vi "MICSD Telem Driver.vi"(0 "VISA Resource Name":refnum<visa-resource-name>="COM3", 1 "Command":T1, 2 "Function":T2(ring)=enum."Transceive (DN -> UP)", 3 "Parameters":string, 5 "error in (no error)":errorcluster, 6 "Target MICS ID":u32=1048576 step=1 format="%.0x", 7 "Transceive Delay mS":dbl=200.0 min=0.0 max=10000.0 step=1.0, 8 "EXID":u32=16773121 step=1 format="%.0x", 9 "CP_DATA IN":u8[](array[numeric]), 10 "RF_Channel":u8=3) -> (13 "CP_DATA OUT":u8[](array[numeric]), 14 "Response Token":string, 15 "Response Code":string, 16 "bChecksum Valid":bool, 17 "tChecksum Valid":bool, 18 "Data":string, 19 "error out":errorcluster)   [LabVIEW 2010]
uses:
  Typedef Command List.ctl
  <vilib>/Utility/file.llb/Write To Spreadsheet File (string).vi
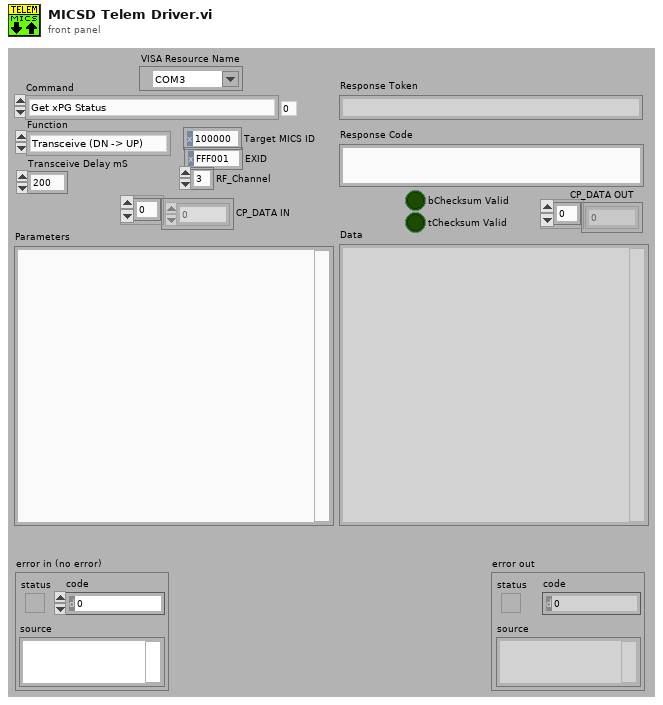
[diagram p1: front panel]
types:
  T1 = typedef "Typedef Command List.ctl" = enum16{"Get xPG Status", "xPG Stimulation", "Select Program", "Increment Program Amplitude", "Decrement Program Amplitude", "Get PoP Constants", "Get PPC Constants", "Get Program Names", "Set Pulse Amplitude", "Increment Pulse Amplitude", "Decrement Pulse Amplitude", "Get Pulse Widths", "Set Pulse Widths", "Increment Pulse Width", "Decrement Pulse Width", "Get Program Frequency", "Set Program Frequency", "Increment Program Frequency", "Decrement Program Frequency", "Inject Event", "Charging Control", "Get xPG Identity", "Set xPG Identity", "Restore Program Defaults", "Get Program Definition", "Set Program Definition", "Get Program Constants", "Set Program Constants", "Get Configurable Device Parameters", "Set Configurable Device Parameters", "Get Pulse Constants", "Set Pulse Constants", "Get Lead Limits", "Set Lead Limits", "Get Channel Calibrations", "Set Channel Calibrations", "<reserved 2>", "<reserved 3>", "<reserved 4>", "<reserved 5>", "<reserved 6>", "<reserved 7>", "Get Stim Asic HV Calibrations", "Set Stim Asic HV Calibrations", "<reserved 8>", "<reserved 9>", "Get CP Data", "Set CP Data", "Clear Log", "Read Log", "Append Log", "Get Patient Program Runtime", "Set Patient Program Runtime", "Impedance Measurement", "Enter Storage Mode", "Echo Short", "Echo Long", "Get General Calibration", "Set General Calibration", "Get Trim List", "Set Trim List", "Get Counter", "Set Counter", "Get Test Stimulation", "Set Test Stimulation", "Get Titration Stimulation", "Set Titration Stimulation", "Get Ramp Time", "Set Ramp Time", "Get VBAT", "Set Software Description Block", "Get Software Description Block", "Write Memory", "Read Memory", "Reset xPG", "Erase Flash Block", "Write Vectors", "Read Vectors", "Diagnostic Data", "Set Background Impedance", "Get Background Impedence ", "Set Test Waveform", "Calibrate Channel", "Get Log Range", "Reserved 0x55", "Reserved 0x56", "MICS Options", "Pair PPC", "Pair POP", "Stop Bootloader", "Tune MICS", "MICS Diagnostics", "Undefined"}
  T2 = enum16{"Open Session", "Close Session", "Downlink Only", "Uplink Only", "Transceive (DN -> UP)"}
  T3 = cluster{"ConfigFlags":u8, "ImplantID":u32, "CompanyID":u8, "Normal_Comm":cluster{"RF_Channel":u8, "UserData":u8, "TX_Mod":u8, "RX_Mod":u8, "RX_BlockSize":u8, "BlockPerPack":u8, "TX_BlockSize":u8}, "Emerg_Comm":cluster{"RF_Channel":u8, "UserData":u8, "TX_Mod":u8, "RX_Mod":u8, "TX_BlockSize":u8, "BlockPerPack":u8, "RX_BlockSize":u8}, "ImplantRev":u8, "245TX_PowerCal":i8, "245TX_Power":i8, "CCA_RSSI_Thresholds":cluster{"ch0":u16, "ch1":u16, "ch2":u16, "ch3":u16, "ch4":u16, "ch5":u16, "ch6":u16, "ch7":u16, "ch8":u16, "ch9":u16}}
  T4 = cluster{"ERROR_OCCURRED":bool, "LINK_STAT_CHANGED":bool, "LINK_QUAL_CHANGED":bool, "400MHZ_TX_ACTIVE":bool, "400MHZ_RX_ACTIVE":bool, "245GHZ_TX_ACTIVE":bool, "DATA_STAT_CHANGED":bool, "SLEEPING":bool, "IDLE":bool, "SEARCHING_FOR_IMPLANT":bool, "STARTING_SESSION":bool, "LISTENING_FOR_EMERG":bool, "IN_SESSION":bool}
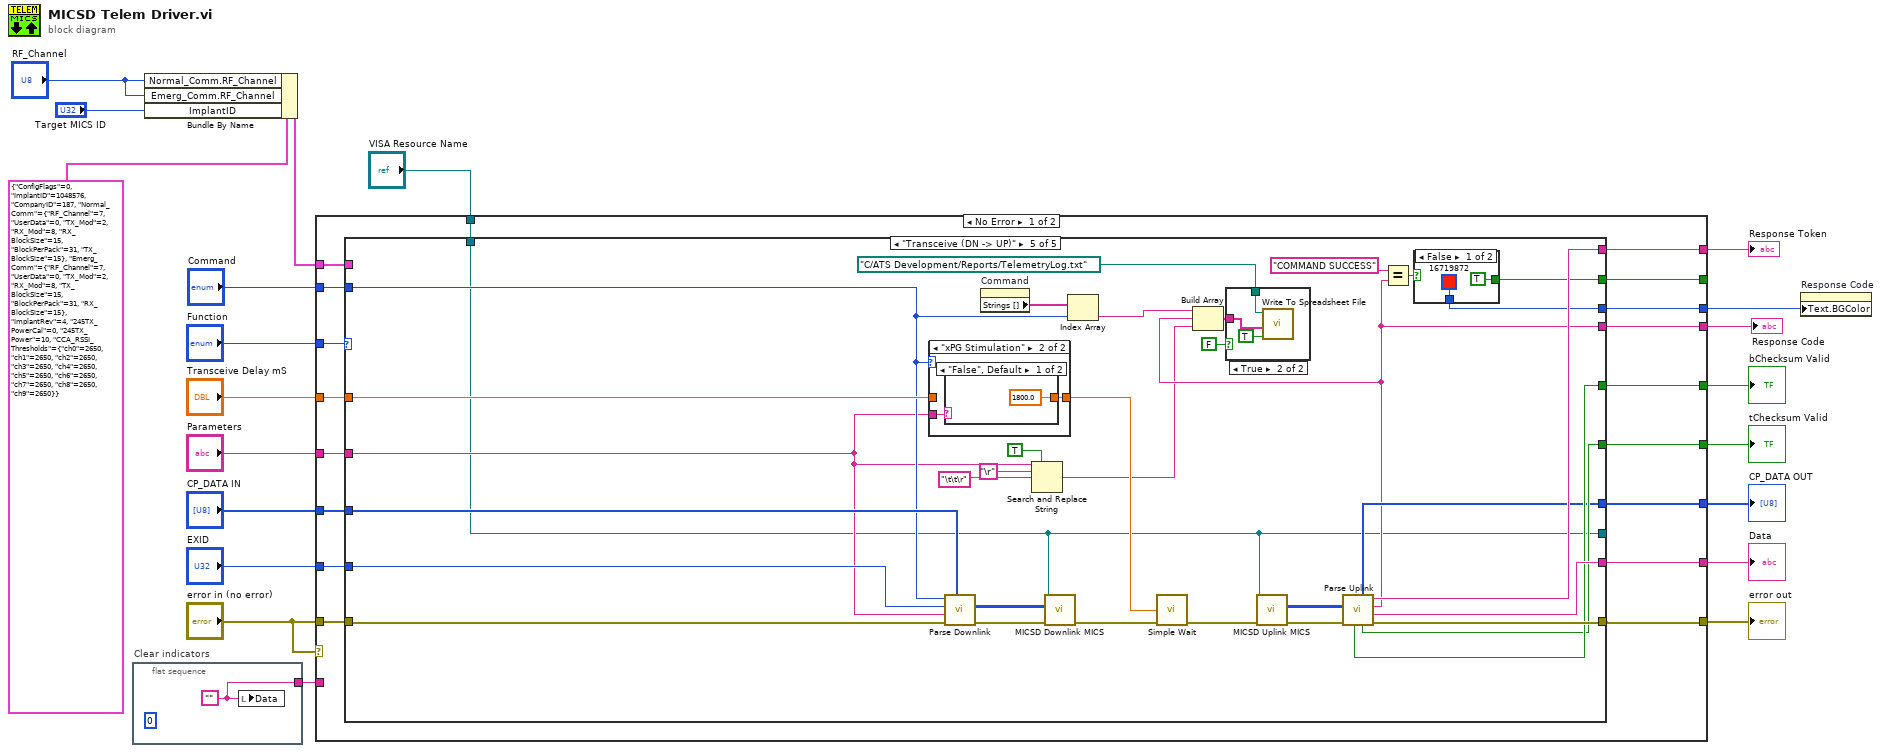
[diagram p0: block diagram]
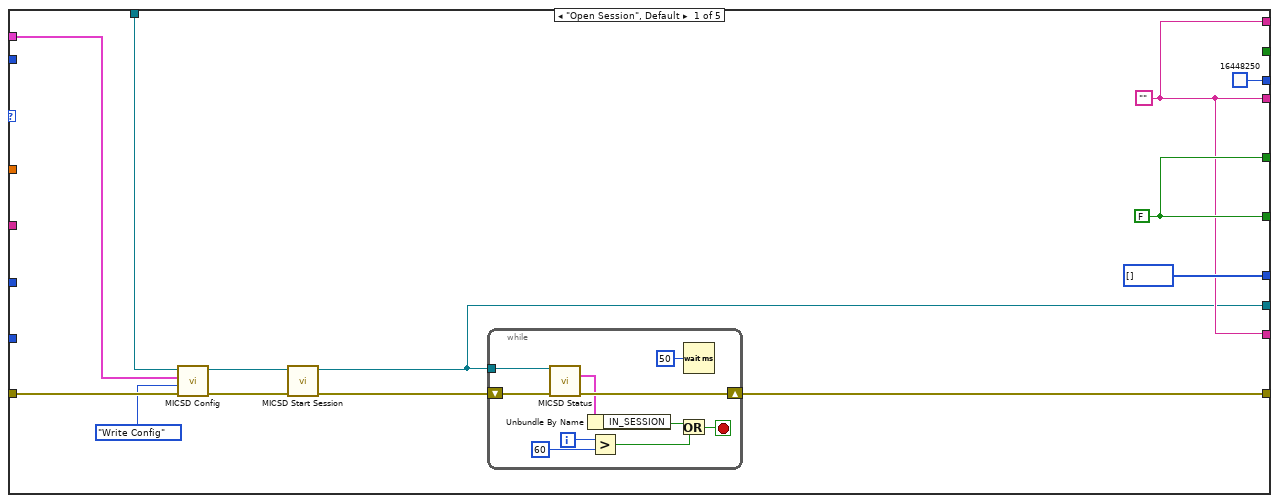
[diagram p2: hidden frame]
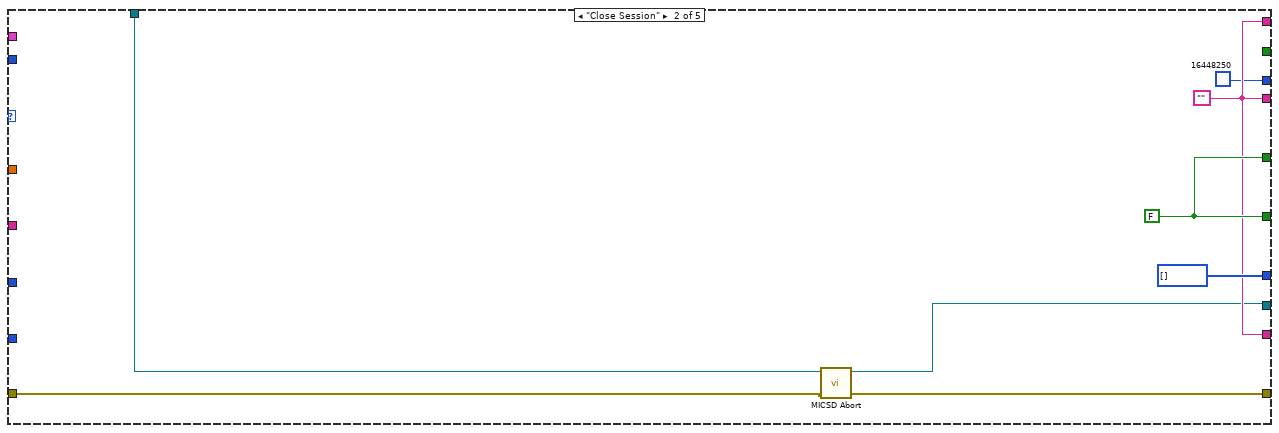
[diagram p3: hidden frame]
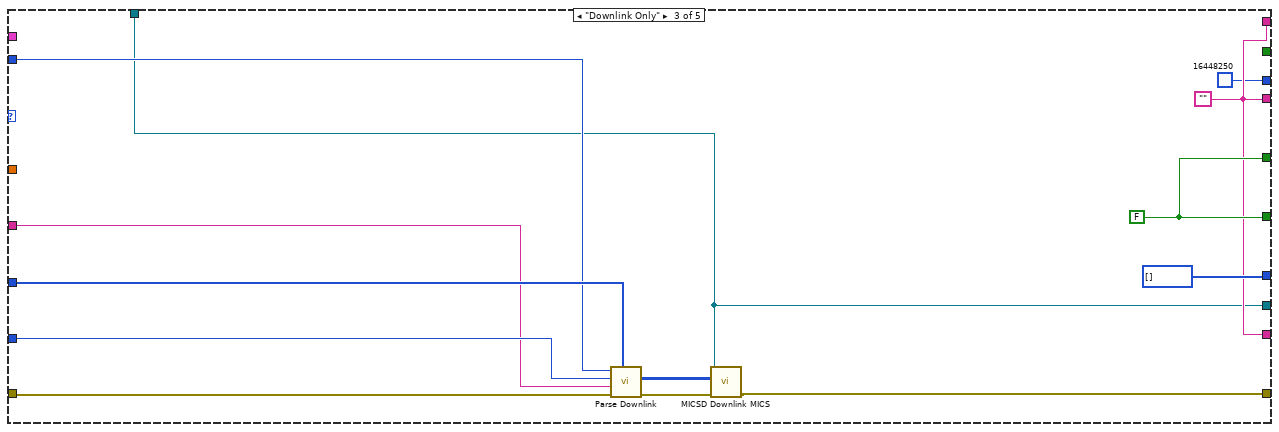
[diagram p4: hidden frame]
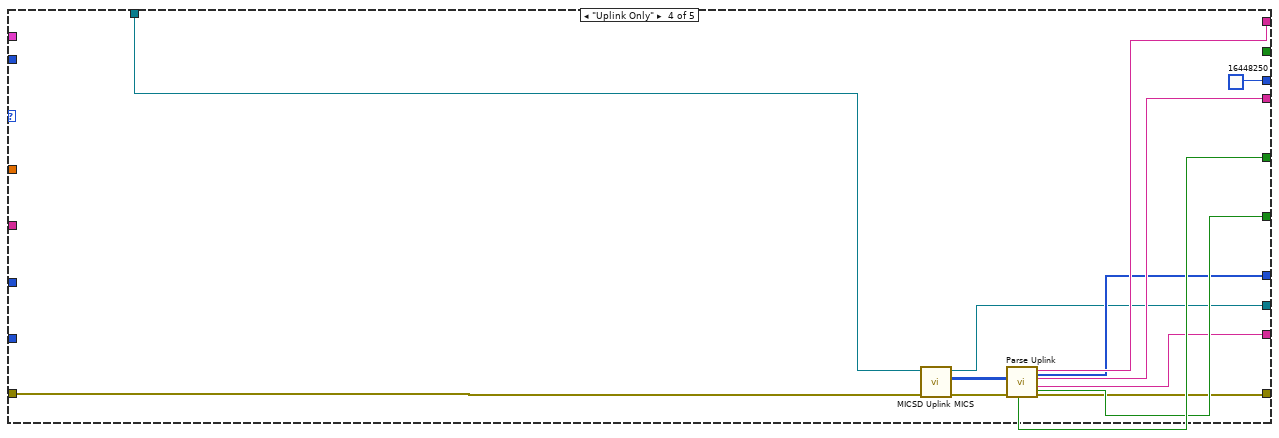
[diagram p5: hidden frame]
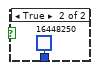
[diagram p6: hidden frame]
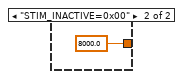
[diagram p9: hidden frame]
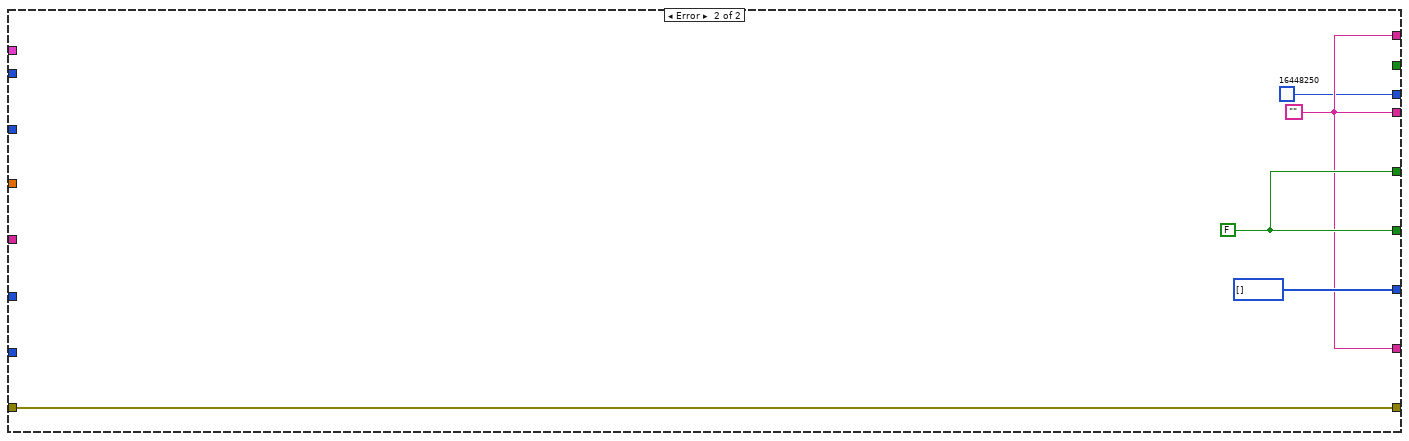
[diagram p10: hidden frame]
diagram:
  n1 = flat-sequence "Clear indicators" {
    tunnel: [w22] -> w15
    frame #0 {
      (unwired) 0 ("Connection Attempt")
      w22 = ""
      n2 = local write "Data"(w22) -> ()
    }
  }
  n3 = Bundle By Name(cluster=T3 {"ConfigFlags"=0, "ImplantID"=1048576, "CompanyID"=187, "Normal_Comm"={"RF_Channel"=7, "UserData"=0, "TX_Mod"=2, "RX_Mod"=8, "RX_BlockSize"=15, "BlockPerPack"=31, "TX_BlockSize"=15}, "Emerg_Comm"={"RF_Channel"=7, "UserData"=0, "TX_Mod"=2, "RX_Mod"=8, "TX_BlockSize"=15, "BlockPerPack"=31, "RX_BlockSize"=15}, "ImplantRev"=4, "245TX_PowerCal"=0, "245TX_Power"=10, "CCA_RSSI_Thresholds"={"ch0"=2650, "ch1"=2650, "ch2"=2650, "ch3"=2650, "ch4"=2650, "ch5"=2650, "ch6"=2650, "ch7"=2650, "ch8"=2650, "ch9"=2650}} ("MICS_Config_In"), "Normal_Comm.RF_Channel"="RF_Channel", "Emerg_Comm.RF_Channel"="RF_Channel", "ImplantID"="Target MICS ID") -> (w14:T3)
  n4 = case shown="No Error" "error in (no error)" {
    tunnel: "error in (no error)" -> [w40 w146]
    tunnel: [w23 w146] -> w12
    tunnel: "Function" -> [w39 _]
    tunnel: "Transceive Delay mS" -> [w32 _]
    tunnel: [w33 w143] -> w6
    tunnel: [w34 w143] -> w7
    tunnel: [w35 w145] -> w8
    tunnel: [w36 w145] -> w9
    tunnel: [w37 u8[] [] ("CP_DATA OUT")] -> w10
    tunnel: [w38 w143] -> w11
    tunnel: "CP_DATA IN" -> [w31 _]
    tunnel: "Command" -> [w30 _]
    tunnel: "EXID" -> [w29 _]
    tunnel: "Parameters" -> [w28 _]
    tunnel: w14 -> [w27 _]
    tunnel: w15 -> [_ _]
    tunnel: [w26 u32 16448250] -> w13
    tunnel: [w25 _] -> _
    tunnel: "VISA Resource Name" -> [w24 _]
    frame No Error {
      n5 = case shown="\"Transceive (DN -> UP)\"" w39 {
        tunnel: w40 -> [w48 w66 w81 w87 w129]
        tunnel: [w42 w65 w73 w90 w125] -> w23
        tunnel: [w44 w68 w74 w91 w124] -> w38
        tunnel: [u8[] [] ("CP_DATA OUT") u8[] [] ("CP_DATA OUT") u8[] [] ("CP_DATA OUT") w92 w120] -> w37
        tunnel: [w52 w69 w76 w93 w121] -> w36
        tunnel: [w52 w69 w76 w94 w122] -> w35
        tunnel: [w44 w68 w74 w95 w109] -> w34
        tunnel: [w44 w68 w74 w96 w123] -> w33
        tunnel: w32 -> [_ _ _ _ w114]
        tunnel: w31 -> [_ _ w79 _ w128]
        tunnel: w30 -> [_ _ w77 _ w111]
        tunnel: w29 -> [_ _ w80 _ w127]
        tunnel: w28 -> [_ _ w78 _ w105]
        tunnel: w27 -> [w43 _ _ _ _]
        tunnel: [u32 16448250 u32 16448250 u32 16448250 u32 16448250 w99] -> w26
        tunnel: [_ _ _ _ w98] -> w25
        tunnel: w24 -> [w49 w64 w71 w85 w97]
        tunnel: [w41 w63 w71 w84 w97] -> _
        frame "Open Session", Default {
          w44 = ""
          w52 = FALSE
          n6 = call "MICSD Config.vi"("error in (no error)"=w48, "Function"=enum16{"Write Config", "Read Config"}."Write Config", "MICS_Config_In"=w43, "VISA Resource Name"=w49) -> ("error out"=w46:errorcluster, "dup VISA Resource Name"=w45:refnum<visa-resource-name>)  [unwired: 5 in, 1 out]
          n7 = call "MICSD Start Session.vi"("error in (no error)"=w46, "VISA Resource Name"=w45) -> ("error out"=w42:errorcluster, "dup VISA Resource Name"=w41:refnum<visa-resource-name>)  [unwired: 8 in]
          n8 = while {
            tunnel: w41 -> [w61]
            shift-right: [w60] -> _
            shift-left: w42 -> [w62]
            i -> [w54]
            stop <- w55 stop-if-true
            n9 = call "MICSD Status.vi"("VISA Resource Name"=w61, "error in (no error)"=w62) -> ("Status Flags"=w59:T4, "error out"=w60:errorcluster)  [unwired: 7 in, 5 out]
            n10 = Unbundle By Name(w59) -> ("IN_SESSION"=w57:bool)
            n11 = Greater?(x=w54, y=60) -> (0:w56:bool)
            n12 = Or(x=w57, y=w56) -> (x .or. y?=w55:bool)
            n13 = Wait (ms)(milliseconds to wait=u32 50) -> ()  [unwired: 1 out]
          }
        }
        frame "Close Session" {
          w68 = ""
          w69 = FALSE
          n14 = call "MICSD Abort.vi"("error in (no error)"=w66, "VISA Resource Name"=w64) -> ("error out"=w65:errorcluster, "dup VISA Resource Name"=w63:refnum<visa-resource-name>)  [unwired: 8 in]
        }
        frame "Downlink Only" {
          w74 = ""
          w76 = FALSE
          n15 = call "Parse Downlink.vi"("CP_DATA IN"=w79, "error in (no error)"=w81, "Parameters"=w78, "EXID"=w80, "Command"=w77) -> ("error out"=w83:errorcluster, "Downlink"=w82:u8[][])  [unwired: 5 in]
          n16 = call "MICSD Downlink MICS.vi"("Error In"=w83, "Downlink"=w82, "VISA Resource Name"=w71) -> ("Error Out"=w73:errorcluster)  [unwired: 7 in, 1 out]
        }
        frame "Uplink Only" {
          n17 = call "MICSD Uplink MICS.vi"("Error In"=w87, "VISA Resource Name"=w85) -> ("Error Out"=w88:errorcluster, "Uplink"=w86:u8[][], "dup VISA Resource Name"=w84:refnum<visa-resource-name>)  [unwired: 7 in]
          n18 = call "Parse Uplink.vi"("error in (no error)"=w88, "Uplink"=w86) -> ("error out"=w90:errorcluster, "Data"=w91:string, "Response Code"=w95:string, "Response Token"=w96:string, "tChecksum Valid"=w93:bool, "CP_DATA"=w92:u8[], "bChecksum Valid"=w94:bool)  [unwired: 3 in]
        }
        frame "Transceive (DN -> UP)" {
          n19 = case shown="\"xPG Stimulation\"" w111 {
            tunnel: w114 -> [w137 _]
            tunnel: [w137 w138] -> w113
            tunnel: w105 -> [_ w139]
            frame "Get xPG Status", Default {
            }
            frame "xPG Stimulation" {
              n20 = case shown="\"False\", Default" w139 {
                tunnel: [1800.0 ("Transceive Delay mS") 8000.0 ("Transceive Delay mS")] -> w138
                frame "False", Default {
                }
                frame "STIM_INACTIVE=0x00" {
                }
              }
            }
          }
          n21 = call "Parse Downlink.vi"("CP_DATA IN"=w128, "error in (no error)"=w129, "Parameters"=w105, "EXID"=w127, "Command"=w111) -> ("error out"=w130:errorcluster, "Downlink"=w118:u8[][])  [unwired: 5 in]
          n22 = property on="Command" class="Enum (strict)"() -> ("Strings []"=w112:string[])  [unwired: 2 in, 2 out]
          n23 = Search and Replace String(replace all?=TRUE ("replace all? (F)"), input string=w105, search string="\r", replace string="\t\t\r" ("search string")) -> (result string=w106:string)  [unwired: 4 in, 3 out]
          n24 = call "MICSD Downlink MICS.vi"("Error In"=w130, "Downlink"=w118, "VISA Resource Name"=w97) -> ("Error Out"=w117:errorcluster)  [unwired: 7 in, 1 out]
          n25 = Index Array(array=w112, index=w111) -> (element=w110:string)
          n26 = call "Simple Wait.vi"("mS"=w113, "error in"=w117) -> ("error out"=w116:errorcluster)  [unwired: 12 in, 1 out]
          n27 = call "MICSD Uplink MICS.vi"("Error In"=w116, "VISA Resource Name"=w97) -> ("Error Out"=w126:errorcluster, "Uplink"=w119:u8[][])  [unwired: 7 in, 1 out]
          n28 = call "Parse Uplink.vi"("error in (no error)"=w126, "Uplink"=w119) -> ("error out"=w125:errorcluster, "Data"=w124:string, "Response Code"=w109:string, "Response Token"=w123:string, "tChecksum Valid"=w121:bool, "CP_DATA"=w120:u8[], "bChecksum Valid"=w122:bool)  [unwired: 3 in]
          n29 = Build Array(w110, w109, w106) -> (w107:string[])
          n30 = case shown="True" FALSE {
            tunnel: path "C:/ATS Development/Reports/TelemetryLog.txt" ("file (use dialog)") -> [_ w136]
            tunnel: w107 -> [_ w135]
            frame False {
            }
            frame True {
              n31 = call-poly <vilib>:"Write To Spreadsheet File.vi"("append to file? (new file:F)"=TRUE, "1D data"=w135, "file path (dialog if empty)"=w136) -> ()  [unwired: 5 in, 1 out]
            }
          }
          n32 = Equal?(x="COMMAND SUCCESS", y=w109) -> (x = y?=w100:bool)
          n33 = case shown="False" w100 {
            tunnel: [u32 16719872 u32 16448250] -> w99
            tunnel: [TRUE _] -> w98
            frame False {
            }
            frame True {
            }
          }
        }
      }
    }
    frame Error {
      w143 = ""
      w145 = FALSE
    }
  }
  "error out" <- w12
  "Response Token" <- w6
  "Response Code" <- w7
  "Data" <- w11
  "CP_DATA OUT" <- w10
  "tChecksum Valid" <- w9
  "bChecksum Valid" <- w8
  n34 = property on="Response Code" class="Str"("Text.BGColor"=w13) -> ()  [unwired: 2 in, 2 out]
